vi "Launch Endpoint Actor.vi"(8 "error in (no error)":errorcluster, 11 "Cobra RT in":refnum<class "Cobra RT.lvclass">) -> (0 "error out":errorcluster, 3 "Cobra RT out":refnum<class "Cobra RT.lvclass">)   [LabVIEW 2019, in "Cobra RT.lvlib" / "Cobra RT.lvclass"]
uses:
  Cobra RT.lvclass
  C:/Program Files (x86)/National Instruments/LabVIEW 2019/vi.lib/ActorFramework/Actor/Actor.lvclass
  <vilib>/NI/Actors/Network Endpoint Actors/Nested Endpoint/Nested Endpoint/Nested Endpoint.lvclass
  C:/Program Files (x86)/National Instruments/LabVIEW 2019/vi.lib/NI/Actors/Network Endpoint Actors/Network Endpoint/Network Endpoint/Network Endpoint.lvclass
  Cobra RT Messages/Endpoint Connected Msg/Endpoint Connected Msg.lvclass
  C:/Program Files (x86)/National Instruments/LabVIEW 2019/vi.lib/NI/Actors/Network Endpoint Actors/Nested Endpoint/Nested Endpoint Messages/Connected Msg/Connected Msg.lvclass
  Cobra RT.lvclass/Cobra RT.ctl
  <vilib>/NI/Actors/Network Endpoint Actors/Network Endpoint/Network Endpoint/Network Endpoint.lvclass/Network Endpoint.ctl
  <vilib>/NI/Actors/Network Endpoint Actors/Nested Endpoint/Nested Endpoint/Nested Endpoint.lvclass/Nested Endpoint.ctl
  <vilib>/NI/Actors/Network Endpoint Actors/Network Endpoint/Network Endpoint/Network Endpoint.lvclass
  <vilib>/ActorFramework/Actor/Actor.lvclass
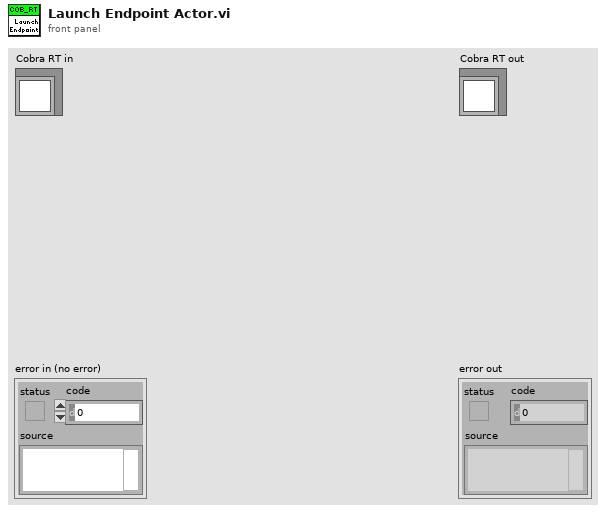
[diagram p1: front panel]
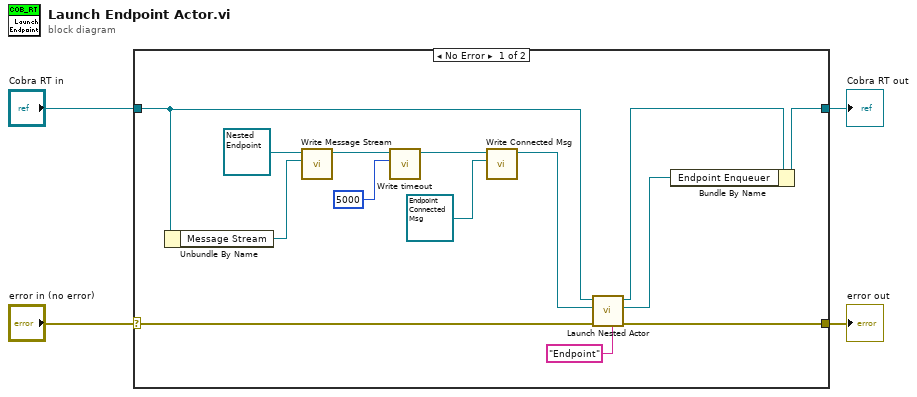
[diagram p0: block diagram]
diagram:
  n1 = case shown="No Error" "error in (no error)" {
    selector: "error in (no error)" -> [w18 w20]
    tunnel: [w17 w20] -> w3
    tunnel: [w8 w19] -> w1
    tunnel: "Cobra RT in" -> [w11 w19]
    frame No Error {
      n2 = Unbundle By Name(w11) -> ("Message Stream"=w14:refnum<class "Message Stream.lvclass">)
      n3 = call <vilib>:"Write Message Stream.vi"("Message Stream"=w14, "Network Endpoint in"=refnum<class "Nested Endpoint.lvclass"> refnum ("Nested Endpoint.lvlib:Nested Endpoint.lvclass")) -> ("Network Endpoint out"=w15:refnum<class "Nested Endpoint.lvclass">)  [unwired: 9 in]
      n4 = call <vilib>:"Write timeout.vi"("timeout"=5000, "Network Endpoint in"=w15) -> ("Network Endpoint out"=w16:refnum<class "Nested Endpoint.lvclass">)  [unwired: 9 in]
      n5 = call <vilib>:"Write Connected Msg.vi"("Nested Endpoint.lvlib:Connected Msg.lvclass"=refnum<class "Endpoint Connected Msg.lvclass"> refnum ("Cobra RT.lvlib:Endpoint Connected Msg.lvclass"), "Nested Endpoint in"=w16) -> ("Nested Endpoint out"=w6:refnum<class "Nested Endpoint.lvclass">)  [unwired: 9 in]
      n6 = call <vilib>:"Launch Nested Actor.vi"("Debug Alias"="Endpoint", "error in (no error)"=w18, "Nested Actor"=w6, "Caller Actor in"=w11) -> ("error out"=w17:errorcluster, "Nested Actor's Enqueuer"=w7:refnum<class "Message Enqueuer.lvclass">, "Caller Actor out"=w9:refnum<class "Cobra RT.lvclass">)  [unwired: 5 in]
      n7 = Bundle By Name(cluster=w9, "Endpoint Enqueuer"=w7) -> (w8:refnum<class "Cobra RT.lvclass">)
    }
    frame Error {
    }
  }
  "error out" <- w3
  "Cobra RT out" <- w1
